vi "Actor Core.vi"(8 "error in":errorcluster, 11 "Master Controller in":refnum<class "EMS User Interface.lvclass">) -> (0 "error out":errorcluster, 3 "Actor out":refnum<class "Actor.lvclass">)   [LabVIEW 2018, in "EMS User Interface Actor.lvlib" / "EMS User Interface.lvclass"]
doc: "(<B>Filename</B>: Actor Framework.lvlib:Actor.lvclass:Actor Core.vi)\n\nReceives messages to the actor, reacts to them, and initiates any error handling that may shut the actor down.\n\nDescendant classes may override this VI to append parallel tasks for the actor to complete while it handles messages. Overrides use the Call Parent Method node."
uses:
  EMS User Interface.lvclass
  C:/Users/Administrator/Desktop/FOR GITHUB UPLOAD/LabVIEW EMS/EMS Generic Actor/EMS Generic/EMS Generic.lvclass
  C:/Program Files (x86)/National Instruments/LabVIEW 2018/vi.lib/ActorFramework/Actor/Actor.lvclass
  <vilib>/ActorFramework/Actor/Actor.lvclass
  Controls/Control Mode Tab Control.ctl
  Controls/Manual Control Tab Control.ctl
  <vilib>/ORNL/CSEISMIC DDS/CSEISMIC DDS Base/Data Types/Controls/Generation Mode.ctl
  <vilib>/ORNL/CSEISMIC DDS/CSEISMIC DDS Base/Data Types/Controls/DeviceID.ctl
  EMS Core/EMS/Controls/Microgrid State.ctl
  Utilities/Status Messaging.llb/Status Message Command.ctl
  EMS Generic Actor/EMS Generic/Controls/Device Information Cluster.ctl
  EMS Generic Actor/EMS Generic/Controls/Device State.ctl
  Controls/Listbox Columns.ctl
  EMS User Interface.lvclass/EMS User Interface.ctl
  <vilib>/ActorFramework/Actor/Actor.lvclass/Actor.ctl
  <vilib>/ActorFramework/Message Enqueuer/Message Enqueuer.lvclass/Message Enqueuer.ctl
  EMS User Interface Messages/Launch Save Status Msg/Launch Save Status Msg.lvclass/Launch Save Status Msg.ctl
  Controls/Dialog Message Selector.ctl
  EMS User Interface Messages/Call Dialog Msg/Call Dialog Msg.lvclass/Call Dialog Msg.ctl
  EMS User Interface Messages/Connect to Device Msg/Connect to Device Msg.lvclass/Connect to Device Msg.ctl
  <vilib>/ORNL/CSEISMIC DDS/CSEISMIC DDS Base/Data Types/DER_Control.ctl
  EMS Core/EMS Messages/Manual Activate Msg/Manual Activate Msg.lvclass/Manual Activate Msg.ctl
  <vilib>/ORNL/CSEISMIC DDS/CSEISMIC DDS Base/Data Types/DER_SetPointP.ctl
  EMS Core/EMS Messages/Manual Real Power Setpoint Msg/Manual Real Power Setpoint Msg.lvclass/Manual Real Power Setpoint Msg.ctl
  <vilib>/ORNL/CSEISMIC DDS/CSEISMIC DDS Base/Data Types/DER_setGenerationMode.ctl
  EMS Core/EMS Messages/Manual Generation Mode Set Msg/Manual Generation Mode Set Msg.lvclass/Manual Generation Mode Set Msg.ctl
  <vilib>/ORNL/CSEISMIC DDS/CSEISMIC DDS Base/Data Types/DER_SetPointQ.ctl
  EMS Core/EMS Messages/Manual Reactive Power Setpoint Msg/Manual Reactive Power Setpoint Msg.lvclass/Manual Reactive Power Setpoint Msg.ctl
  <vilib>/Utility/miscctls.llb/LVRowAndColumnTypeDef.ctl
  <vilib>/ORNL/CSEISMIC DDS/CSEISMIC DDS Base/Data Types/IED_Status.ctl
  <vilib>/ORNL/CSEISMIC DDS/CSEISMIC DDS Base/Data Types/Controls/Timestamp.ctl
  <vilib>/ORNL/CSEISMIC DDS/CSEISMIC DDS Base/Data Types/DER_Measurement.ctl
  <vilib>/ORNL/CSEISMIC DDS/CSEISMIC DDS Base/Data Types/SmartRelay_Measurement.ctl
  <vilib>/ORNL/CSEISMIC DDS/CSEISMIC DDS Base/Data Types/DER_Status.ctl
  <vilib>/ORNL/CSEISMIC DDS/CSEISMIC DDS Base/Data Types/Controls/DroopCurve.ctl
  <vilib>/Analysis/1siggen.llb/Ramp Pattern by Samples.vi
  <vilib>/ActorFramework/Message Enqueuer/Init from Existing Queue.vi
  <vilib>/ActorFramework/Message Enqueuer/Enqueue.vi
  EMS User Interface Messages/Reset Configuration Msg/Reset Configuration Msg.lvclass
  C:/Program Files (x86)/National Instruments/LabVIEW 2018/vi.lib/ActorFramework/Message/Message.lvclass
  EMS User Interface Messages/Launch Save Configuration Msg/Launch Save Configuration Msg.lvclass
  EMS User Interface Messages/Launch Load Configuration Msg/Launch Load Configuration Msg.lvclass
  <vilib>/ActorFramework/Stop Msg/Stop Msg.lvclass
  EMS User Interface Messages/Launch Save Status Msg/Launch Save Status Msg.lvclass
  EMS User Interface Messages/Set Default Configuration Msg/Set Default Configuration Msg.lvclass
  EMS User Interface Messages/Launch Devices to Load Dialog Msg/Launch Devices to Load Dialog Msg.lvclass
  EMS User Interface Messages/Launch VF Device Selection Dialog Msg/Launch VF Device Selection Dialog Msg.lvclass
  EMS User Interface Messages/Call Dialog Msg/Call Dialog Msg.lvclass
  EMS User Interface Messages/Automatic EMS Msg/Automatic EMS Msg.lvclass
  EMS User Interface Messages/Manual EMS Msg/Manual EMS Msg.lvclass
  EMS User Interface Messages/Start EMS Msg/Start EMS Msg.lvclass
  EMS User Interface Messages/Execute EMS Msg/Execute EMS Msg.lvclass
  EMS User Interface Messages/Transition EMS Msg/Transition EMS Msg.lvclass
  EMS User Interface Messages/Connect to Device Msg/Connect to Device Msg.lvclass
  EMS Core/EMS Messages/Manual Activate Msg/Manual Activate Msg.lvclass
  EMS Core/EMS Messages/Manual Real Power Setpoint Msg/Manual Real Power Setpoint Msg.lvclass
  EMS Core/EMS Messages/Manual Generation Mode Set Msg/Manual Generation Mode Set Msg.lvclass
  EMS Core/EMS Messages/Manual Reactive Power Setpoint Msg/Manual Reactive Power Setpoint Msg.lvclass
  Global Variables/Global Variables.vi
  <vilib>/ActorFramework/Message Priority Queue/Priority Enqueue.vi
  <vilib>/ActorFramework/Message Enqueuer/Message Enqueuer.lvclass
  EMS Generic Actor/EMS Generic/EMS Generic.lvclass
  EMS Core/EMS/EMS.lvclass
  Utilities/Status Messaging.llb/Status Messaging.lvlib
  <vilib>/ORNL/CSEISMIC DDS/CSEISMIC DDS Base/CSEISMIC DDS.lvclass
  Utilities/Password Protection/Password Protection.lvlib
  <vilib>/Analysis/NI_AALBase.lvlib
panel:
  out "DevIDs in Config":T1[](array[typedef])
  in  "Control Mode":T2
  out "Current Status Bool":bool
  out "Current State":string
  out "Current Status":string
  in  "Transition":bool
  in  "Execution":bool
  in  "Start":bool
  out "Status":string
  out "Devices":i32(listbox)
  in  "Connect":bool
  out "Manual Status":string
  in  "Device Connect":T3
  in  "Activate Device?":bool caption="Activate\nDevice?"
  in  "Write Mode":bool caption="Write\nMode"
  in  "Write Q":bool
  in  "Write P":bool
  in  "Q Setpoint (kVAR)":dbl(slide) scale=0.0..330.0
  in  "P Setpoint (kW)":dbl(slide) scale=0.0..330.0 scale format="%#.6g"
  in  "Write Activation":bool caption="Write\nActivation"
  out "P Meas":dbl[](array[numeric])
  out "Q Meas":dbl[](array[numeric])
  in  "Gen Mode":T4=enum."PQ"
  out "Active":bool
  out "Inactive":bool
  in  "Channels":i32[](listbox)
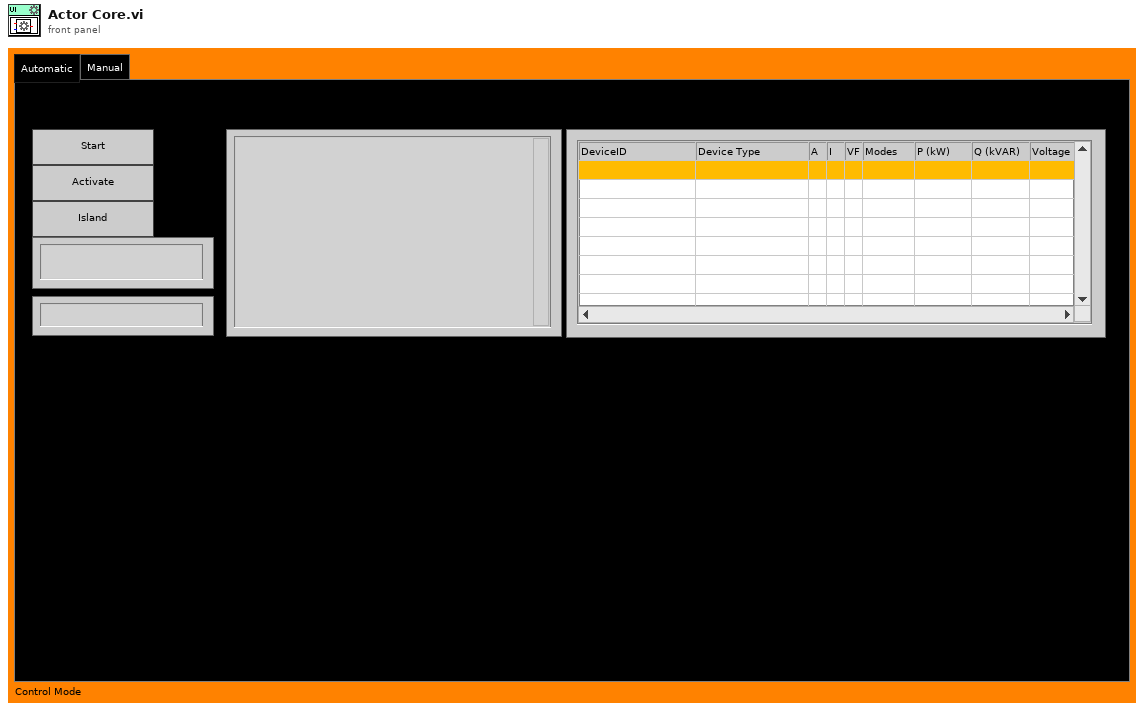
[diagram p1: front panel]
types:
  T1 = typedef "CSEISMIC DDS.lvlib/CSEISMIC DDS.lvclass/DeviceID.ctl" = string
  T2 = typedef "EMS User Interface Actor.lvlib/EMS User Interface.lvclass/Control Mode Tab Control.ctl" = enum32{"Automatic", "Manual"}
  T3 = typedef "EMS User Interface Actor.lvlib/EMS User Interface.lvclass/Manual Control Tab Control.ctl" = enum32{"Off", "Standard"}
  T4 = typedef "CSEISMIC DDS.lvlib/CSEISMIC DDS.lvclass/Generation Mode.ctl" = enum32{"Invalid", "PQ", "Droop", "PV", "PF", "VF"}
  T5 = typedef "EMS User Interface Actor.lvlib/EMS User Interface.lvclass/Listbox Columns.ctl" = cluster{"DeviceID Column":i32, "Device Type Column":i32, "Active Column":i32, "Inactive Column":i32, "VF Column":i32, "Modes Column":i32, "P_Total Column":i32, "Q_Total Column":i32, "V_Avg Column":i32, "I_Total Column":i32, "Frequency Column":i32, "P_A Column":i32, "P_B Column":i32, "P_C Column":i32, "Q_A Column":i32, "Q_B Column":i32, "Q_C Column":i32, "V_A Column":i32, "V_B Column":i32, "V_C Column":i32, "I_A Column":i32, "I_B Column":i32, "I_C Column":i32}
  T6 = typedef "EMS Generic Actor.lvlib/EMS Generic.lvclass/Device Information Cluster.ctl" = cluster{"Device State":T7, "data":variant}
  T7 = typedef "EMS Generic Actor.lvlib/EMS Generic.lvclass/Device State.ctl" = enum16{"Invalid", "Clear", "DevIDs in Config", "DevIDs on uGrid", "DevIDs not on uGrid", "Update IED_Status", "Update DER_Status", "Update DER_Measurement", "Update SmartRelay_Measurement"}
  T8 = enum32{"Invalid", "Standard", "Closed", "Hidden", "Minimized", "Maximized"}
  T9 = typedef "Status Messaging.lvlib/Status Message Command.ctl" = enum16{"Write", "Obtain", "Kill"}
  T10 = typedef "EMS Core.lvlib/EMS.lvclass/Microgrid State.ctl" = enum16{"Discovery", "Commissioning", "Activation", "Blackstart", "OnGrid", "OffGrid", "Island", "Resynchronization", "Manual", "Shutdown", "Stop"}
  T11 = typedef "EMS User Interface Actor.lvlib/EMS User Interface.lvclass/Master Controller User Events.ctl" = cluster{"Current State":refnum<user-event>, "Current Status":refnum<user-event>, "Device List":refnum<user-event>, "P Meas":refnum<user-event>, "Q Meas":refnum<user-event>, "P Set Max":refnum<user-event>, "Q Set Max":refnum<user-event>, "IED_Status":refnum<user-event>, "Device State Information":refnum<user-event>}
  T12 = typedef "EMS User Interface Actor.lvlib/EMS User Interface.lvclass/Dialog Message Selector.ctl" = enum16{"Nominal Voltage", "Nominal Frequency", "Optimization Parameters"}
  T13 = typedef "CSEISMIC DDS.lvlib/CSEISMIC DDS.lvclass/DER_Control.ctl" = cluster{"DeviceID":T1, "Activate":bool, "Deactivate":bool}
  T14 = typedef "CSEISMIC DDS.lvlib/CSEISMIC DDS.lvclass/DER_SetPointP.ctl" = cluster{"DeviceID":T1, "RealPower (kW)":dbl[]}
  T15 = typedef "CSEISMIC DDS.lvlib/CSEISMIC DDS.lvclass/DER_setGenerationMode.ctl" = cluster{"DeviceID":T1, "Mode":T4}
  T16 = typedef "CSEISMIC DDS.lvlib/CSEISMIC DDS.lvclass/DER_SetPointQ.ctl" = cluster{"DeviceID":T1, "ReactivePower (kVAR)":dbl[]}
  T17 = enum8{"Enabled", "Disabled", "Disabled and Grayed Out"}
  T18 = typedef "LVRectTypeDef.ctl" = cluster{"Left":i16, "Top":i16, "Right":i16, "Bottom":i16}
  T19 = typedef "LVRowAndColumnTypeDef.ctl" = cluster{"Row":i32, "Column":i32}
  T20 = typedef "CSEISMIC DDS.lvlib/CSEISMIC DDS.lvclass/IED_Status.ctl" = cluster{"DeviceID":T1, "Timestamp":T21, "MicrogridID":u8, "Active":bool, "Inactive":bool, "Error":i32, "Fault":bool, "ErrorString":string}
  T21 = typedef "CSEISMIC DDS.lvlib/CSEISMIC DDS.lvclass/Timestamp.ctl" = cluster{"Seconds":u64, "Remainder":u64}
  T22 = typedef "CSEISMIC DDS.lvlib/CSEISMIC DDS.lvclass/DER_Measurement.ctl" = cluster{"DeviceID":T1, "Voltage":dbl[], "Current":dbl[], "RealPower":dbl[], "ReactivePower":dbl[], "LineConfig":u8[], "Frequency":dbl}
  T23 = typedef "CSEISMIC DDS.lvlib/CSEISMIC DDS.lvclass/SmartRelay_Measurement.ctl" = cluster{"DeviceID":T1, "PrimaryVoltage":dbl[], "SecondaryVoltage":dbl[], "Current":dbl[], "RealPower":dbl[], "ReactivePower":dbl[], "LineConfig":u8[], "Frequency":dbl}
  T24 = typedef "CSEISMIC DDS.lvlib/CSEISMIC DDS.lvclass/DER_Status.ctl" = cluster{"DeviceID":T1, "VFControl":bool, "PControl":bool, "QControl":bool, "PFControl":bool, "PVControl":bool, "Droop":bool, "Unbalanced":bool, "MicrogridVF":bool, "RealDroop(kW)":T25, "ReactiveDroop(kVar)":T25}
  T25 = typedef "CSEISMIC DDS.lvlib/CSEISMIC DDS.lvclass/DroopCurve.ctl" = cluster{"XMin":dbl, "XMax":dbl, "YMin":dbl, "YMax":dbl}
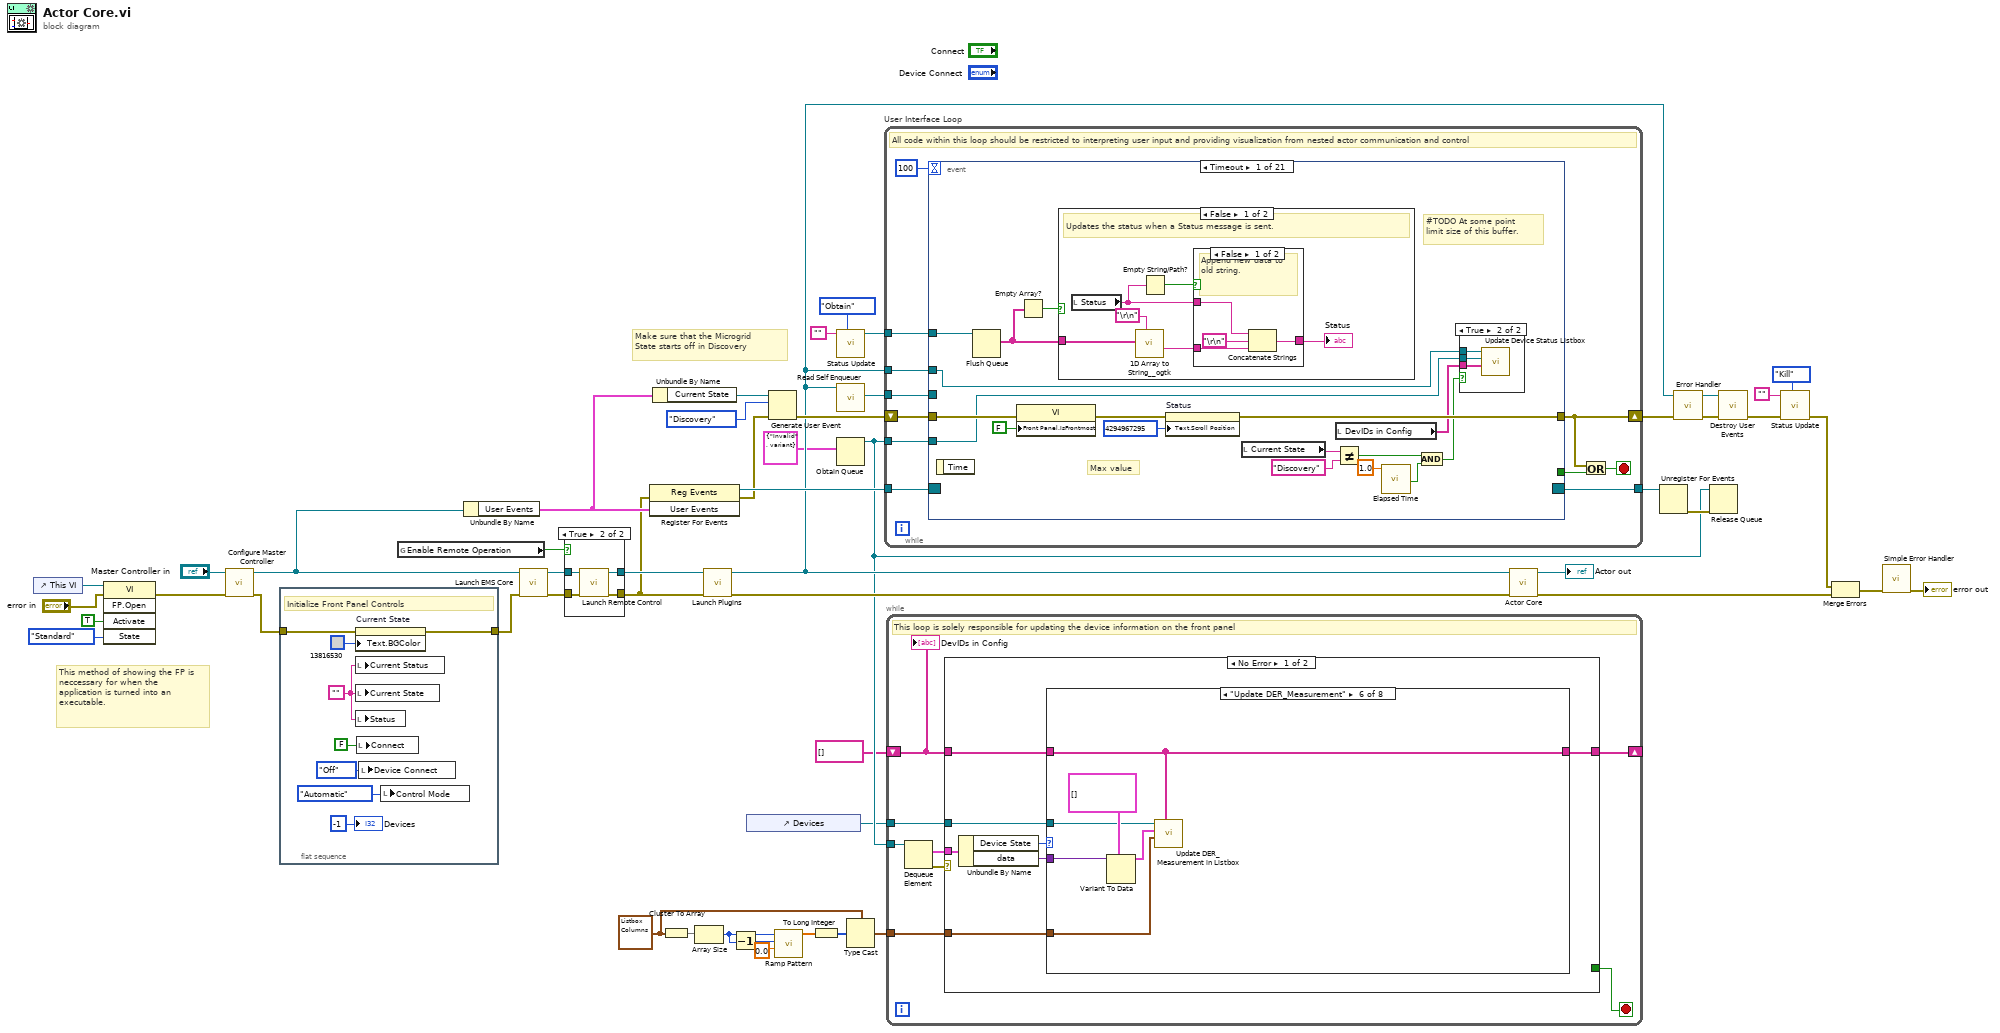
[diagram p0: block diagram]
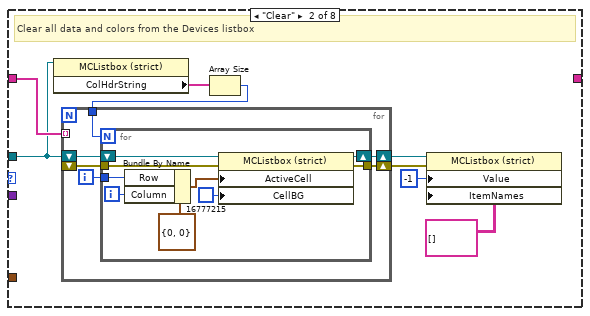
[diagram p3: hidden frame]
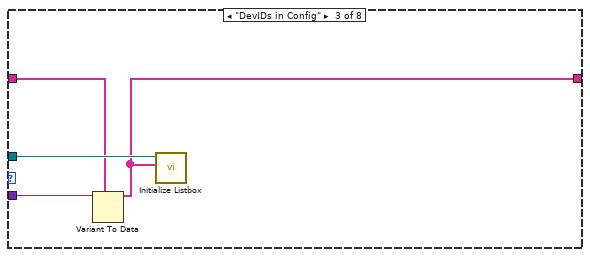
[diagram p4: hidden frame]
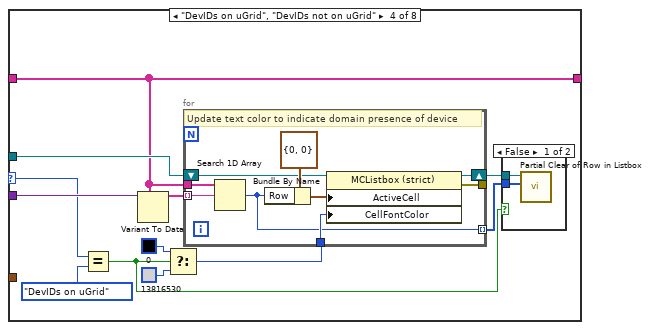
[diagram p5: hidden frame]
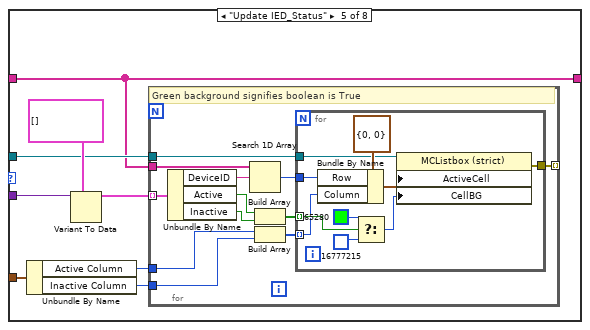
[diagram p7: hidden frame]
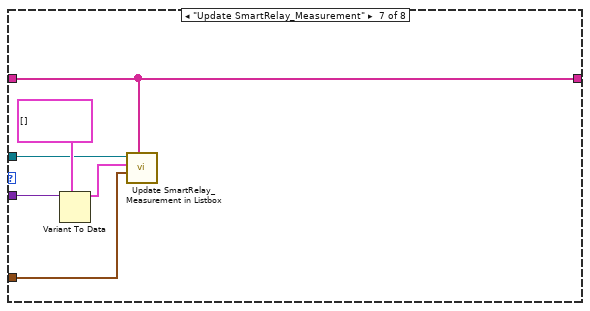
[diagram p8: hidden frame]
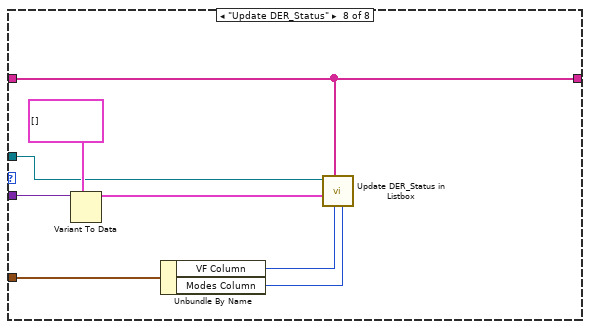
[diagram p9: hidden frame]
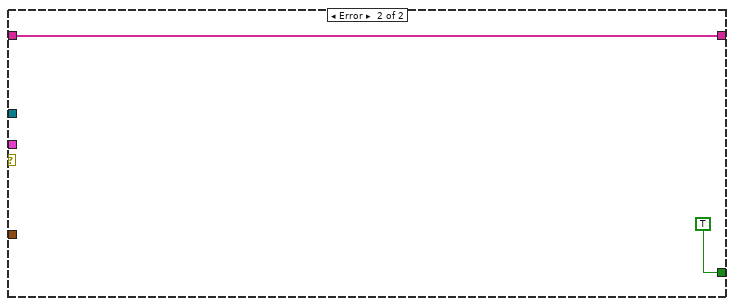
[diagram p10: hidden frame]
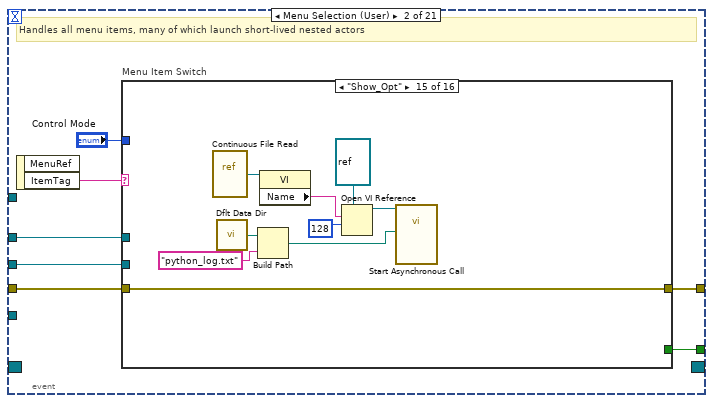
[diagram p15: hidden frame]
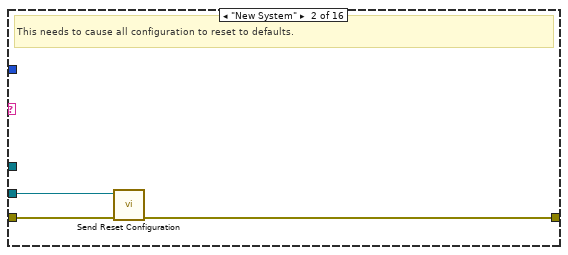
[diagram p17: hidden frame]
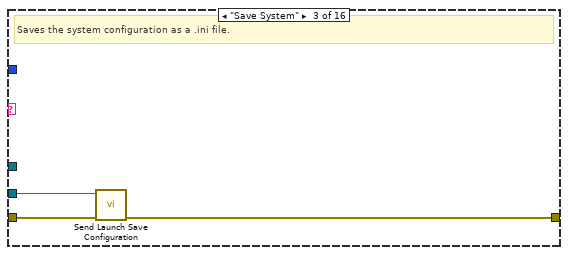
[diagram p18: hidden frame]
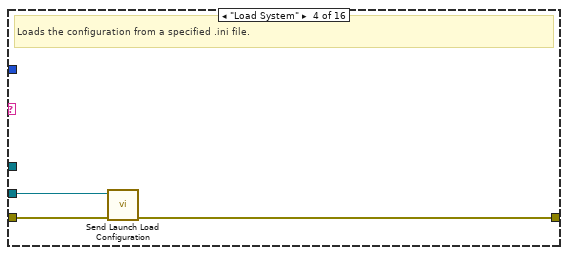
[diagram p19: hidden frame]
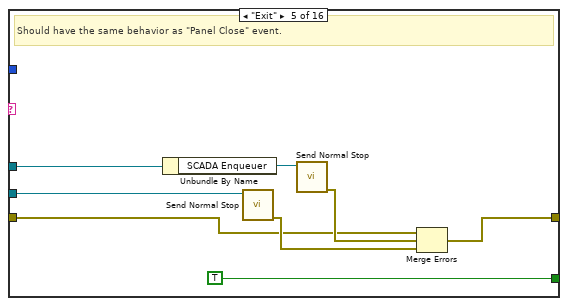
[diagram p20: hidden frame]
diagram:
  w1 = T5 {"DeviceID Column"=0, "Device Type Column"=0, "Active Column"=0, "Inactive Column"=0, "VF Column"=0, "Modes Column"=0, "P_Total Column"=0, "Q_Total Column"=0, "V_Avg Column"=0, "I_Total Column"=0, "Frequency Column"=0, "P_A Column"=0, "P_B Column"=0, "P_C Column"=0, "Q_A Column"=0, "Q_B Column"=0, "Q_C Column"=0, "V_A Column"=0, "V_B Column"=0, "V_C Column"=0, "I_A Column"=0, "I_B Column"=0, "I_C Column"=0} ("DER_Meas Listbox Columns")
  # "Make sure that the Microgrid State starts off in Discovery"
  # "This method of showing the FP is neccessary for when the application is turned into an executable."
  n1 = control-ref of="This VI"() -> (w34:refnum<vi>)
  n2 = invoke class="VI" method="FP.Open"(reference=w34, error in="error in", "Activate"=TRUE ("Activate?"), "State"=T8."Standard") -> (error out=w30:errorcluster)  [unwired: 1 in, 4 out]
  n3 = call "Configure Master Controller.vi"("error in"=w30, "EMS Generic in"="Master Controller in") -> ("error out"=w41:errorcluster, "EMS Generic out"=w42:refnum<class "EMS User Interface.lvclass">)  [unwired: 8 in]
  n4 = flat-sequence {
    tunnel: w41 -> [w57]
    tunnel: [w56] -> w47
    frame #0 {
      w59 = ""
      # "Initialize Front Panel Controls"
      n5 = property on="Current State" class="Str"(error in=w57, "Text.BGColor"=u32 13816530) -> (error out=w56:errorcluster)  [unwired: 1 in, 1 out]
      n6 = local write "Current Status"(w59) -> ()
      n7 = local write "Current State"(w59) -> ()
      n8 = local write "Status"(w59) -> ()
      n9 = local write "Connect"(FALSE ("Connect")) -> ()
      n10 = local write "Device Connect"(Manual_Control_Tab_Control."Off" ("Device Connect")) -> ()
      n11 = local write "Control Mode"(Control_Mode_Tab_Control."Automatic" ("Control Mode")) -> ()
      "Devices" <- -1 ("Devices")
    }
  }
  n12 = global read "Global Variables.vi" "Enable Remote Operation"() -> (w18:bool)
  n13 = Unbundle By Name(w42) -> ("User Events"=w45:T11)
  n14 = call "Launch EMS Core.vi"("error in"=w47, "Master Controller in"=w42) -> ("error out"=w19:errorcluster, "Master Controller out"=w20:refnum<class "EMS User Interface.lvclass">)  [unwired: 8 in]
  n15 = case shown="True" w18 {
    tunnel: w20 -> [w61 w65]
    tunnel: [w61 w64] -> w17
    tunnel: w19 -> [w60 w63]
    tunnel: [w60 w62] -> w16
    frame False {
    }
    frame True {
      n16 = call "Launch Remote Control.vi"("error in"=w63, "Master Controller in"=w65) -> ("error out"=w62:errorcluster, "Master Controller out"=w64:refnum<class "EMS User Interface.lvclass">)  [unwired: 8 in]
    }
  }
  n17 = register-events(error in=w16, w45) -> (reference out=w50:refnum<event-registration>, error out=w46:errorcluster)  [unwired: 1 in]
  n18 = Unbundle By Name(w45) -> ("Current State"=w44:refnum<user-event>)
  n19 = Cluster To Array(cluster=w1) -> (array=w5:i32[])
  n20 = Array Size(array=w5) -> (size(s)=w6:i32)
  n21 = call "Launch Plugins.vi"("error in"=w16, "Master Controller in"=w17) -> ("error out"=w14:errorcluster, "Master Controller out"=w15:refnum<class "EMS User Interface.lvclass">)  [unwired: 8 in]
  n22 = Decrement(x=w6) -> (x-1=w8:i32)
  n23 = control-ref of="Devices"() -> (w10:refnum<vi>)
  n24 = Generate User Event(user event=w44, event data cluster=Microgrid_State."Discovery" ("event data"), error in=w46) -> (error out=w27:errorcluster)  [unwired: 1 in, 1 out]
  n25 = call-poly <vilib>:"Ramp Pattern.vi"("start"=0.0, "end"=w8, "samples"=w6) -> ("Ramp Pattern"=w4:dbl[])  [unwired: 7 in, 1 out]
  n26 = To Long Integer(number=w4) -> (32bit integer=w3:i32[])
  n27 = call "Status Update.vi"("Command (Write)"=Status_Message_Command."Obtain", "Status Update"="") -> ("queue out"=w38:refnum<queue>)  [unwired: 8 in, 1 out]
  n28 = call <vilib>:"Read Self Enqueuer.vi"("Actor"=w15) -> ("Self Enqueuer"=w48:refnum<class "Message Enqueuer.lvclass">)  [unwired: 10 in]
  n29 = Obtain Queue(element data type=T6 {"Device State"=enum."Invalid", "data"=variant} ("Device State Information")) -> (queue out=w11:refnum<queue>)  [unwired: 4 in, 2 out]
  n30 = Type Cast(type=w1, x=w3) -> (*(type *) &x=w2:T5)
  n31 = while "User Interface Loop" {
    shift-right: [w69] -> w23
    shift-left: w27 -> [w76]
    tunnel: w50 -> [w75]
    tunnel: [w74] -> w49
    tunnel: w48 -> [w73]
    tunnel: w38 -> [w72]
    tunnel: w15 -> [w70]
    tunnel: w11 -> [w66]
    stop <- w67 stop-if-true
    # "All code within this loop should be restricted to interpreting user input and providing visualization from nested actor communication and control"
    n32 = event shown="[0] Timeout" {
      selector: w75 -> [_ _ _ _ _ _ _ _ _ _ _ _ _ _ _ _ _ _ _ _ _]
      dyn-events: [_ _ _ _ _ _ _ _ _ _ _ _ _ _ _ _ _ _ _ _ _] -> w74
      timeout: 100 -> [_ _ _ _ _ _ _ _ _ _ _ _ _ _ _ _ _ _ _ _ _]
      tunnel: w76 -> [w92 w112 w210 w213 w222 w230 w238 w274 w292 w313 w330 _ w360 _ w491 _ _ w506 w510 _ w516]
      tunnel: [w93 w111 w209 w212 w223 w229 w237 w273 w291 w312 w329 _ w362 _ w478 _ _ w505 w508 _ w513] -> w69
      tunnel: [_ w110 _ _ _ _ _ _ _ _ _ _ _ _ _ _ _ _ _ _ TRUE ("Discard?")] -> w68
      tunnel: w73 -> [_ w113 w211 w214 w224 w231 w239 _ _ _ _ _ _ _ _ _ _ _ _ _ w517]
      tunnel: w72 -> [w91 _ _ _ _ _ _ _ _ _ _ _ _ _ _ _ _ _ _ _ _]
      tunnel: w70 -> [w83 w108 _ _ _ _ _ w272 w293 w314 w328 _ w357 _ _ _ _ _ _ _ w519]
      tunnel: w66 -> [w84 _ _ _ _ _ _ _ _ _ _ w350 w356 _ _ _ _ _ _ _ _]
      event Timeout {
        # "Max value"
        # "#TODO At some point limit size of this buffer."
        n33 = event-data() -> ()  [unwired: 1 in, 1 out]
        n34 = Flush Queue(queue=w91) -> (remaining elements=w87:string[])  [unwired: 1 in, 2 out]
        n35 = property class="VI"(error in=w92, "Front Panel.IsFrontmost"=FALSE ("Front Panel Window:Is Frontmost")) -> (error out=w89:errorcluster)  [unwired: 1 in, 1 out]
        n36 = Empty Array?(array=w87) -> (empty?=w86:bool)
        n37 = case shown="False" w86 {
          tunnel: w87 -> [w99 _]
          frame False {
            # "Updates the status when a Status message is sent."
            n38 = local read "Status"() -> (w100:string)
            n39 = call <userlib>:"1D Array to String__ogtk.vi"("delimiter (Tab)"="\r\n", "Array of Strings"=w99) -> ("delimited string"=w97:string)  [unwired: 9 in]
            n40 = Empty String/Path?(string/path=w100) -> (empty?=w101:bool)
            n41 = case shown="False" w101 {
              tunnel: [w106 w107] -> w102
              tunnel: w97 -> [w105 w107]
              tunnel: w100 -> [w103 _]
              frame False {
                # "Append new data to old string."
                n42 = Concatenate Strings(w103, "\r\n", w105) -> (w106:string)
              }
              frame True {
                # "Set new data as string."
              }
            }
            "Status" <- w102
          }
          frame True {
          }
        }
        n43 = property on="Status" class="Str"(error in=w89, "Text.Scroll Position"=u32 4294967295) -> (error out=w93:errorcluster)  [unwired: 1 in, 1 out]
        n44 = local read "Current State"() -> (w81:string)
        n45 = local read "DevIDs in Config"() -> (w82:T1[])
        n46 = Not Equal?(x=w81, y="Discovery") -> (x != y?=w79:bool)
        n47 = call "Elapsed Time"("Time Target (s)"=1.0) -> ("Time has Elapsed"=w78:bool)  [unwired: 11 in, 7 out]
        n48 = And(x=w79, y=w78) -> (x .and. y?=w77:bool)
        n49 = case shown="True" w77 {
          tunnel: w84 -> [_ w96]
          tunnel: w83 -> [_ w95]
          tunnel: w82 -> [_ w94]
          frame False {
          }
          frame True {
            n50 = call "Update Device Status Listbox.vi"("DeviceIDs"=w94, "queue in"=w96, "EMS User Interface in"=w95) -> ()  [unwired: 9 in]
          }
        }
      }
      event Menu Selection (User) {
        # "Handles all menu items, many of which launch short-lived nested actors"
        n51 = event-data() -> ("ItemTag"=w114:string)  [unwired: 1 in, 1 out]
        n52 = case "Menu Item Switch" shown="\"Show_Opt\"" w114 {
          tunnel: w113 -> [_ w118 w119 w123 w126 w134 _ w141 w144 w147 w149 w153 w156 w176 _ w205]
          tunnel: w112 -> [w115 w117 w121 w124 w128 w136 w138 w140 w143 w146 w151 w155 w160 w180 w204 w207]
          tunnel: [w115 w116 w120 w122 w127 w135 w138 w139 w142 w145 w150 w154 w159 w179 w204 w206] -> w111
          tunnel: [_ _ _ _ TRUE ("Discard?") _ _ _ _ _ _ _ _ _ _ _] -> w110
          tunnel: "Control Mode" -> [_ _ _ _ _ _ _ _ _ _ _ _ w158 w178 _ _]
          tunnel: w108 -> [_ _ _ _ w125 _ _ _ _ _ _ _ _ _ _ _]
          frame "False", Default {
            # "Do nothing for unconfigured menu items"
          }
          frame "New System" {
            # "This needs to cause all configuration to reset to defaults."
            n53 = call "Send Reset Configuration.vi"("error in (no error)"=w117, "Message Enqueuer"=w118) -> ("error out"=w116:errorcluster)  [unwired: 8 in, 1 out]
          }
          frame "Save System" {
            # "Saves the system configuration as a .ini file."
            n54 = call "Send Launch Save Configuration.vi"("error in (no error)"=w121, "Message Enqueuer"=w119) -> ("error out"=w120:errorcluster)  [unwired: 8 in, 1 out]
          }
          frame "Load System" {
            # "Loads the configuration from a specified .ini file."
            n55 = call "Send Launch Load Configuration.vi"("error in (no error)"=w124, "Message Enqueuer"=w123) -> ("error out"=w122:errorcluster)  [unwired: 8 in, 1 out]
          }
          frame "Exit" {
            # "Should have the same behavior as \"Panel Close\" event."
            n56 = Unbundle By Name(w125) -> ("SCADA Enqueuer"=w129:refnum<class "Message Enqueuer.lvclass">)
            n57 = call <vilib>:"Send Normal Stop.vi"("Message Enqueuer"=w126) -> ("error out"=w131:errorcluster)  [unwired: 10 in]
            n58 = call <vilib>:"Send Normal Stop.vi"("Message Enqueuer"=w129) -> ("error out"=w130:errorcluster)  [unwired: 10 in]
            n59 = Merge Errors(w128, w130, w131) -> (w127:errorcluster)
          }
          frame "Save Status History" {
            # "Saves the Status text box to a text file."
            n60 = local read "Status"() -> (w133:string)
            n61 = call "Send Launch Save Status.vi"("error in (no error)"=w136, "Status"=w133, "Message Enqueuer"=w134) -> ("error out"=w135:errorcluster)  [unwired: 7 in, 1 out]
          }
          frame "Clear Status History" {
            # "Clears the Status text box."
            n62 = local write "Status"("") -> ()
          }
          frame "DEFAULT" {
            # "Set the current configuration file as the default configuration file."
            n63 = call "Send Set Default Configuration.vi"("error in (no error)"=w140, "Message Enqueuer"=w141) -> ("error out"=w139:errorcluster)  [unwired: 8 in, 1 out]
          }
          frame "Devices to Load" {
            # "Launches a dialog box that allows the user to choose which available device to use in the system."
            n64 = call "Send Launch Devices to Load Dialog.vi"("error in (no error)"=w143, "Message Enqueuer"=w144) -> ("error out"=w142:errorcluster)  [unwired: 8 in, 1 out]
          }
          frame "V/F Device" {
            # "Launches a dialog box that allows the user to choose which available device to use in the system."
            n65 = call "Send Launch VF Device Selection Dialog.vi"("error in (no error)"=w146, "Message Enqueuer"=w147) -> ("error out"=w145:errorcluster)  [unwired: 8 in, 1 out]
          }
          frame "Nominal Frequency" {
            # "Launch a subactor to set the nominal frequency"
            n66 = call "Send Call Dialog.vi"("error in (no error)"=w151, "Dialog"=Dialog_Message_Selector."Nominal Frequency", "Message Enqueuer"=w149) -> ("error out"=w150:errorcluster)  [unwired: 7 in, 1 out]
          }
          frame "Nominal Voltage" {
            # "Launches a subactor to set Nominal Voltage"
            n67 = call "Send Call Dialog.vi"("error in (no error)"=w155, "Dialog"=Dialog_Message_Selector."Nominal Voltage", "Message Enqueuer"=w153) -> ("error out"=w154:errorcluster)  [unwired: 7 in, 1 out]
          }
          frame "Automatic" {
            # "Change the visible area and window position for Automatic Control Mode"
            n68 = case shown="\"Manual\"" w158 {
              tunnel: w160 -> [w161 w164]
              tunnel: [w161 w170] -> w159
              tunnel: w156 -> [_ w165]
              frame "Automatic", Default {
                # "If it's already Automatic/Normal, do nothing"
              }
              frame "Manual" {
                # "Make sure that the current control mode is Manual"
                n69 = control-ref of="This VI"() -> (w166:refnum<vi>)
                n70 = call "Send Automatic EMS.vi"("error in (no error)"=w164, "Message Enqueuer"=w165) -> ("error out"=w163:errorcluster)  [unwired: 8 in, 1 out]
                n71 = property class="VI"(reference=w166, error in=w163) -> (reference out=w169:refnum<vi>, error out=w171:errorcluster, "Front Panel.PanelBounds"=w168:T18)
                n72 = in-place {
                  n73 = in-place-cluster #1(w168) -> ("Right"=w175:i16)
                  n74 = Add(x=w175, y=i16 -25) -> (x+y=w173:i16)
                  n75 = in-place-cluster #1("Right"=w173) -> (w167:T18)
                }
                n76 = local read "Connect"() -> (w162:bool)
                n77 = case shown="True" w162 {
                  frame False {
                  }
                  frame True {
                    n78 = property on="Connect" class="Bool (strict)"("Val(Sgnl)"=FALSE ("Connect")) -> ()  [unwired: 2 in, 2 out]
                  }
                }
                n79 = property class="VI"(reference=w169, error in=w171, "Front Panel.PanelBounds"=w167) -> (error out=w170:errorcluster)  [unwired: 1 out]
              }
            }
            n80 = local write "Control Mode"(Control_Mode_Tab_Control."Automatic" ("Control Mode")) -> ()
          }
          frame "Manual" {
            # "Change the visible area and window position for Manual Control Mode"
            n81 = case shown="\"Automatic\"" w178 {
              tunnel: w180 -> [w185 w195]
              tunnel: [w190 w195] -> w179
              tunnel: w176 -> [w186 _]
              frame "Automatic" {
                # "Make sure that the current control mode is Normal/Automatic. Adjust the window width bigger and send the message to put the EMS into the Stop state if neccessary."
                n82 = control-ref of="This VI"() -> (w183:refnum<vi>)
                n83 = call "Send Manual EMS.vi"("error in"=w185, "Message Enqueuer"=w186) -> ("error out"=w184:errorcluster)  [unwired: 8 in, 1 out]
                n84 = local write "Connect"(FALSE ("Connect")) -> ()
                n85 = local write "Manual Status"("") -> ()
                n86 = property class="VI"(reference=w183, error in=w184) -> (reference out=w189:refnum<vi>, error out=w191:errorcluster, "Front Panel.PanelBounds"=w188:T18)
                n87 = in-place {
                  n88 = in-place-cluster #2(w188) -> ("Right"=w194:i16)
                  n89 = Add(x=w194, y=i16 25) -> (x+y=w192:i16)
                  n90 = in-place-cluster #2("Right"=w192) -> (w187:T18)
                }
                n91 = property class="VI"(reference=w189, error in=w191, "Front Panel.PanelBounds"=w187) -> (error out=w190:errorcluster)  [unwired: 1 out]
              }
              frame "Manual", Default {
                # "If it's already Manual, do nothing"
              }
            }
            n92 = local write "Control Mode"(Control_Mode_Tab_Control."Manual" ("Control Mode")) -> ()
          }
          frame "Show_Opt" {
            n93 = vi-ref "Continuous File Read.vi"() -> (w197:refnum<vi>)
            n94 = call <vilib>:"Dflt Data Dir.vi"() -> ("App:Default Data Directory"=w203:path)
            n95 = Build Path(base path=w203, name or relative path="python_log.txt") -> (appended path=w198:path)
            n96 = property class="VI"(reference=w197) -> ("Name"=w196:string)  [unwired: 1 in, 2 out]
            n97 = Open VI Reference(type specifier VI Refnum (for type only)=refnum<vi> refnum, vi path=w196, options=128) -> (vi reference=w199:refnum<vi>)  [unwired: 3 in, 1 out]
            n98 = call-by-ref "Start Asynchronous Call"(reference=w199, "file path"=w198) -> ()  [unwired: 11 in, 3 out]
          }
          frame "Opt_Params" {
            n99 = call "Send Call Dialog.vi"("error in (no error)"=w207, "Dialog"=Dialog_Message_Selector."Optimization Parameters", "Message Enqueuer"=w205) -> ("error out"=w206:errorcluster)  [unwired: 7 in, 1 out]
          }
        }
      }
      event "Start": Value Change {
        # "React to a vlaue change in the START button. This is context-specific and reacts differently based on the Microgrid state"
        n100 = event-data() -> ()  [unwired: 1 in, 1 out]
        n101 = call "Send Start EMS.vi"("error in (no error)"=w210, "Message Enqueuer"=w211) -> ("error out"=w209:errorcluster)  [unwired: 8 in, 1 out]
      }
      event "Execution": Value Change {
        # "React to a vlaue change in the EXECUTION button. This is context-specific and reacts differently based on the Microgrid state"
        n102 = event-data() -> ()  [unwired: 1 in, 1 out]
        n103 = call "Send Execute EMS.vi"("error in (no error)"=w213, "Message Enqueuer"=w214) -> ("error out"=w212:errorcluster)  [unwired: 8 in, 1 out]
      }
      event "Transition": Value Change {
        # "React to a vlaue change in the TRANSITION button. This is context-specific and reacts differently based on the Microgrid state"
        n104 = event-data() -> ()  [unwired: 1 in, 1 out]
        n105 = call <vilib>:"Application Directory.vi"() -> ("Application Directory"=w218:path)
        n106 = Build Path(base path=w218, name or relative path="Configuration") -> (appended path=w217:path)
        n107 = Build Path(base path=w217, name or relative path="EMS-config.ini") -> (appended path=w215:path)
        n108 = call "Password Protection.vi"("error in"=w222, "configuration file path"=w215) -> ("error out"=w221:errorcluster, "Validated?"=w220:bool)  [unwired: 8 in]
        n109 = case shown="True" w220 {
          tunnel: w224 -> [_ w228]
          tunnel: [w225 w227] -> w223
          tunnel: w221 -> [w225 w226]
          frame False {
          }
          frame True {
            n110 = call "Send Transition EMS.vi"("error in (no error)"=w226, "Message Enqueuer"=w228) -> ("error out"=w227:errorcluster)  [unwired: 8 in, 1 out]
          }
        }
      }
      event "Channels": Value Change {
        # "Solely for disconnecting the last device when it is either deselected or another device is selected"
        n111 = event-data() -> ()  [unwired: 1 in, 1 out]
        n112 = local read "Connect"() -> (w232:bool)
        n113 = case "Device Connected?" shown="True" w232 {
          tunnel: w231 -> [_ _]
          tunnel: w230 -> [w233 w236]
          tunnel: [w233 w235] -> w229
          frame False {
            # "Not connected to anything, so do nothing."
          }
          frame True {
            # "Disconnect device, we use the value change (signaling) to execute the event case for Connect Value Change."
            n114 = property on="Connect" class="Bool (strict)"(error in=w236, "Val(Sgnl)"=FALSE ("Connect")) -> (error out=w235:errorcluster)  [unwired: 1 in, 1 out]
          }
        }
      }
      event "Connect": Value Change {
        # "Connect to selected device, making a link to bringing back measurements, status, and info and allowing setting setpoints"
        n115 = event-data() -> ("NewVal"=w241:bool)  [unwired: 1 in]
        n116 = case "Connect Device?" shown="True" w241 {
          tunnel: "Channels" -> [_ w262]
          tunnel: w239 -> [w246 w260]
          tunnel: w238 -> [w245 w261]
          tunnel: [w244 w259] -> w237
          frame False {
            # "Disconnect the device. This should put the Microgrid into the Stop state, that will move into Device Discovery."
            n117 = call "Send Start EMS.vi"("error in (no error)"=w245, "Message Enqueuer"=w246) -> ("error out"=w244:errorcluster)  [unwired: 8 in, 1 out]
            n118 = local write "Manual Status"("") -> ()
            n119 = local write "Device Connect"(Manual_Control_Tab_Control."Off" ("Device Connect Tab")) -> ()
          }
          frame True {
            # "hide certain controls when manual device is PCC"
            # "Connect to the device. This puts SCADA and the Microgird into a Manual Control State"
            n120 = for {
              tunnel: w262 -> [w265] mode=indexing
              shift-right: [w267] -> _
              shift-left: w260 -> [w269]
              shift-right: [w268] -> w259
              shift-left: w261 -> [w270]
              tunnel: [w263] -> w253 mode=indexing
              # "For now, this should only run once"
              n121 = property on="Channels" class="MCListbox (strict)"() -> ("ItemNames"=w266:string[][])  [unwired: 2 in, 2 out]
              n122 = Index Array(array=w266, index (row)=w265, index (col)=3 ("disabled index (col)")) -> (element=w263:string)
              n123 = call "Send Connect to Device.vi"("error in (no error)"=w270, "DeviceID"=w263, "Message Enqueuer"=w269) -> ("error out"=w268:errorcluster, "Message Enqueuer out"=w267:refnum<class "Message Enqueuer.lvclass">)  [unwired: 7 in]
            }
            n124 = call "Determine Device Types.vi"("DeviceIDs"=w253) -> ("Device Classes"=w252:string[])  [unwired: 9 in]
            n125 = call <userlib>:"1D Array to String__ogtk.vi"("delimiter (Tab)"=",", "Array of Strings"=w253) -> ("delimited string"=w255:string)  [unwired: 9 in]
            n126 = Format Into String(format string="Connected: %s", w255) -> (resulting string=→"Manual Status":string)  [unwired: 2 in, 1 out]
            n127 = Search 1D Array(1D array=w252, element="PCC") -> (index of element=w250:i32)  [unwired: 1 in]
            n128 = Less Than 0?(x=w250) -> (x < 0?=w248:bool)
            n129 = local write "Device Connect"(Manual_Control_Tab_Control."Standard" ("Device Connect Tab")) -> ()
            n130 = control-ref of="This VI"() -> (w249:refnum<vi>)
            n131 = call "Set Visibility of Select Manual Controls.vi"("Visible (F)"=w248, "Control Names"=string[] ["P Setpoint (kW)", "Write P", "Write Mode", "Gen Mode", "Write Q", "Q Setpoint (kVAR)"], "VI in"=w249) -> ()  [unwired: 9 in]
          }
        }
      }
      event "Write Activation": Value Change {
        # "#TODO Move some of this code into a message to make sure it only runs while the microgrid is in manual mode"
        # "This event should only execute if the Microgrid is in Manual Mode and a Device is connected"
        n132 = event-data() -> ()  [unwired: 1 in, 1 out]
        n133 = local read "Device Connect"() -> (w275:T3)
        n134 = case "Device Connection Status?" shown="\"Standard\"" w275 {
          tunnel: w274 -> [w276 w287]
          tunnel: [w276 w286] -> w273
          tunnel: w272 -> [_ w289]
          tunnel: "Activate Device?" -> [_ w277]
          frame "Off", Default {
            # "do nothing"
          }
          frame "Standard" {
            # "Only allow activation or deactivation of device while connected"
            n135 = Unbundle By Name(w289) -> ("SCADA Enqueuer"=w288:refnum<class "Message Enqueuer.lvclass">)
            n136 = property on="Channels" class="MCListbox (strict)"() -> ("ItemNames"=w283:string[][], "Value"=w284:i32[])  [unwired: 2 in, 2 out]
            n137 = Index Array(array=w284) -> (element=w285:i32)  [unwired: 1 in]
            n138 = Index Array(array=w283, index (row)=w285, index (col)=3 ("disabled index (col)")) -> (element=w280:string)
            n139 = Not(x=w277) -> (.not. x?=w278:bool)
            n140 = Bundle By Name(cluster=T13 {"DeviceID"="", "Activate"=FALSE, "Deactivate"=FALSE} ("DER_Control"), "Activate"=w277, "Deactivate"=w278, "DeviceID"=w280) -> (w279:T13)
            n141 = call "Send Manual Activate.vi"("error in (no error)"=w287, "DER_Control"=w279, "Message Enqueuer"=w288) -> ("error out"=w286:errorcluster)  [unwired: 7 in, 1 out]
          }
        }
      }
      event "Write P": Value Change {
        # "#TODO Move some of this code into a message to make sure it only runs while the microgrid is in manual mode"
        # "Manually send a Real Power setpoint to the connected device."
        n142 = event-data() -> ()  [unwired: 1 in, 1 out]
        n143 = local read "Device Connect"() -> (w290:T3)
        n144 = case "Device Connection Status" shown="\"Standard\"" w290 {
          tunnel: w293 -> [_ w299]
          tunnel: w292 -> [w294 w296]
          tunnel: [w294 w295] -> w291
          frame "Off", Default {
            # "Do nothing"
          }
          frame "Standard" {
            # "Turn the single setpoint into a 3-phase setpoint, take the active DeviceID and send the message"
            n145 = Unbundle By Name(w299) -> ("SCADA Enqueuer"=w298:refnum<class "Message Enqueuer.lvclass">)
            n146 = property on="Channels" class="MCListbox (strict)"() -> ("ItemNames"=w308:string[][], "Value"=w309:i32[])  [unwired: 2 in, 2 out]
            n147 = Index Array(array=w309) -> (element=w310:i32)  [unwired: 1 in]
            n148 = Divide(x="P Setpoint (kW)", y=3.0) -> (x/y=w303:dbl)
            n149 = Initialize Array(w303, 3 ("dimension size")) -> (w300:dbl[])
            n150 = Index Array(array=w308, index (row)=w310, index (col)=3 ("disabled index (col)")) -> (element=w301:string)
            n151 = Bundle By Name(cluster=T14 {"DeviceID"="", "RealPower (kW)"=[]} ("DER_SetPointP"), "RealPower (kW)"=w300, "DeviceID"=w301) -> (w297:T14)
            n152 = call "Send Manual Real Power Setpoint.vi"("error in (no error)"=w296, "DER_SetPointP"=w297, "Message Enqueuer"=w298) -> ("error out"=w295:errorcluster)  [unwired: 7 in, 1 out]
          }
        }
      }
      event "Write Mode": Value Change {
        # "#TODO Move some of this code into a message to make sure it only runs while the microgrid is in manual mode"
        # "Manually send a Real Power setpoint to the connected device."
        n153 = event-data() -> ()  [unwired: 1 in, 1 out]
        n154 = local read "Device Connect"() -> (w311:T3)
        n155 = case "Device Connection Status" shown="\"Standard\"" w311 {
          tunnel: w314 -> [_ w321]
          tunnel: w313 -> [w315 w316]
          tunnel: [w315 w317] -> w312
          frame "Off", Default {
            # "Do nothing"
          }
          frame "Standard" {
            # "Turn the single setpoint into a 3-phase setpoint, take the active DeviceID and send the message"
            n156 = Unbundle By Name(w321) -> ("SCADA Enqueuer"=w318:refnum<class "Message Enqueuer.lvclass">)
            n157 = property on="Channels" class="MCListbox (strict)"() -> ("ItemNames"=w325:string[][], "Value"=w326:i32[])  [unwired: 2 in, 2 out]
            n158 = Index Array(array=w326) -> (element=w327:i32)  [unwired: 1 in]
            n159 = Index Array(array=w325, index (row)=w327, index (col)=3 ("disabled index (col)")) -> (element=w322:string)
            n160 = Bundle By Name(cluster=T15 {"DeviceID"="", "Mode"=enum."Invalid"} ("DER_setGenerationMode"), "Mode"="Gen Mode", "DeviceID"=w322) -> (w319:T15)
            n161 = call "Send Manual Generation Mode Set.vi"("error in (no error)"=w316, "DER_setGenerationMode"=w319, "Message Enqueuer"=w318) -> ("error out"=w317:errorcluster)  [unwired: 7 in, 1 out]
          }
        }
      }
      event "Write Q": Value Change {
        # "#TODO Move some of this code into a message to make sure it only runs while the microgrid is in manual mode"
        # "Set the reactive power setpoint under connected condition"
        n162 = event-data() -> ()  [unwired: 1 in, 1 out]
        n163 = local read "Device Connect"() -> (w331:T3)
        n164 = case "Device Connection Status?" shown="\"Standard\"" w331 {
          tunnel: w330 -> [w332 w335]
          tunnel: [w332 w334] -> w329
          tunnel: w328 -> [_ w337]
          frame "Off", Default {
            # "Do nothing"
          }
          frame "Standard" {
            # "The device is connected, allow the message to go through"
            n165 = property on="Channels" class="MCListbox (strict)"() -> ("ItemNames"=w346:string[][], "Value"=w347:i32[])  [unwired: 2 in, 2 out]
            n166 = Unbundle By Name(w337) -> ("SCADA Enqueuer"=w336:refnum<class "Message Enqueuer.lvclass">)
            n167 = Index Array(array=w347) -> (element=w348:i32)  [unwired: 1 in]
            n168 = Divide(x="Q Setpoint (kVAR)", y=3.0) -> (x/y=w342:dbl)
            n169 = Initialize Array(w342, 3 ("dimension size")) -> (w339:dbl[])
            n170 = Index Array(array=w346, index (row)=w348, index (col)=3 ("disabled index (col)")) -> (element=w340:string)
            n171 = Bundle By Name(cluster=T16 {"DeviceID"="", "ReactivePower (kVAR)"=[]} ("DER_SetPointQ"), "ReactivePower (kVAR)"=w339, "DeviceID"=w340) -> (w333:T16)
            n172 = call "Send Manual Reactive Power Setpoint.vi"("error in (no error)"=w335, "DER_SetPointQ"=w333, "Message Enqueuer"=w336) -> ("error out"=w334:errorcluster)  [unwired: 7 in, 1 out]
          }
        }
      }
      event User Event {
        n173 = event-data() -> ("Device State"=w352:T7, "data"=w351:variant)  [unwired: 1 in]
        n174 = Bundle By Name(cluster=T6 {"Device State"=enum."Invalid", "data"=variant} ("Device State Information"), "Device State"=w352, "data"=w351) -> (w349:T6)
        n175 = Enqueue Element(queue=w350, element=w349) -> ()  [unwired: 2 in, 3 out]
      }
      event User Event {
        # "Handles changes in front panel objects during changes of state."
        n176 = event-data() -> ("Microgrid State"=w355:T10)  [unwired: 1 in]
        n177 = Format Into String(error in=w360, w355) -> (resulting string=→"Current State":string, error out=w359:errorcluster)  [unwired: 2 in]
        n178 = feedback-in #3(w355) -> ()
        n179 = feedback #3() -> (w354:T10)  [unwired: 1 in]
        n180 = case "Microgrid States Switch Statement" shown="\"Discovery\"" w355 {
          tunnel: [u32 16776960 u32 16776960 u32 16744448 u32 255 u32 65280 u32 16711680 u32 8454016 u32 16744576 u32 16776960 u32 16776960 u32 0] -> w361
          tunnel: w359 -> [w373 w383 w401 w413 w423 w436 w445 w455 w464 w473 w476]
          tunnel: [w375 w385 w399 w411 w416 w434 w443 w453 w462 w471 w476] -> w358
          tunnel: w357 -> [_ _ _ _ w417 w428 _ _ _ _ _]
          tunnel: w356 -> [w366 _ _ _ _ _ _ _ _ _ _]
          tunnel: w355 -> [_ _ w395 _ _ _ _ _ _ _ _]
          tunnel: w354 -> [_ _ w394 _ _ _ _ _ _ _ _]
          frame "Discovery" {
            w367 = T17."Disabled and Grayed Out" ("Disabled")
            n181 = Enqueue Element(queue=w366, element=T6 {"Device State"=enum."Clear", "data"=variant}) -> ()  [unwired: 2 in, 3 out]
            n182 = property on="Execution" class="Bool"(error in=w373, "DisabledEnum"=w367, "BoolText.Text"="") -> (error out=w374:errorcluster)  [unwired: 1 in, 1 out]
            n183 = property on="Transition" class="Bool"(error in=w374, "DisabledEnum"=w367, "BoolText.Text"="") -> (error out=w372:errorcluster)  [unwired: 1 in, 1 out]
            n184 = property on="Current Status Bool" class="Bool (strict)"("BoolText.Text"="") -> ()  [unwired: 2 in, 2 out]
            n185 = property on="Start" class="Bool"(error in=w372, "DisabledEnum"=T17."Enabled" ("Disabled"), "BoolText.Text"="Start" ("Boolean Text.Text")) -> (error out=w375:errorcluster)  [unwired: 1 in, 1 out]
          }
          frame "Commissioning" {
            w377 = T17."Disabled and Grayed Out" ("Disabled")
            n186 = property on="Execution" class="Bool"(error in=w383, "DisabledEnum"=w377, "BoolText.Text"="") -> (error out=w384:errorcluster)  [unwired: 1 in, 1 out]
            n187 = property on="Transition" class="Bool"(error in=w384, "DisabledEnum"=w377, "BoolText.Text"="") -> (error out=w382:errorcluster)  [unwired: 1 in, 1 out]
            n188 = property on="Start" class="Bool"(error in=w382, "DisabledEnum"=T17."Enabled" ("Disabled"), "BoolText.Text"="Stop" ("Boolean Text.Text")) -> (error out=w385:errorcluster)  [unwired: 1 in, 1 out]
          }
          frame "Activation" {
            w391 = T17."Disabled and Grayed Out" ("Disabled")
            # "Prevent people from clicking Activate more than once"
            n189 = Equal?(x=w395, y=w394) -> (x = y?=w390:bool)
            n190 = Select(t="", s=w390, f="Activate" ("Boolean Text.Text")) -> (s? t:f=w387:string)
            n191 = Select(t=w391, s=w390, f=T17."Enabled" ("Disabled")) -> (s? t:f=w392:T17)
            n192 = property on="Execution" class="Bool"(error in=w401, "DisabledEnum"=w392, "BoolText.Text"=w387) -> (error out=w402:errorcluster)  [unwired: 1 in, 1 out]
            n193 = property on="Transition" class="Bool"(error in=w402, "DisabledEnum"=w391, "BoolText.Text"="") -> (error out=w400:errorcluster)  [unwired: 1 in, 1 out]
            n194 = property on="Start" class="Bool"(error in=w400, "DisabledEnum"=T17."Enabled" ("Disabled"), "BoolText.Text"="Stop" ("Boolean Text.Text")) -> (error out=w399:errorcluster)  [unwired: 1 in, 1 out]
          }
          frame "Blackstart" {
            n195 = property on="Execution" class="Bool"(error in=w413, "DisabledEnum"=T17."Enabled" ("Disabled"), "BoolText.Text"="Blackstart" ("Boolean Text.Text")) -> (error out=w414:errorcluster)  [unwired: 1 in, 1 out]
            n196 = property on="Transition" class="Bool"(error in=w414, "DisabledEnum"=T17."Disabled and Grayed Out" ("Disabled"), "BoolText.Text"="") -> (error out=w412:errorcluster)  [unwired: 1 in, 1 out]
            n197 = property on="Start" class="Bool"(error in=w412, "DisabledEnum"=T17."Enabled" ("Disabled"), "BoolText.Text"="Stop" ("Boolean Text.Text")) -> (error out=w411:errorcluster)  [unwired: 1 in, 1 out]
          }
          frame "OffGrid" {
            w418 = T17."Enabled" ("Disabled")
            n198 = property on="Execution" class="Bool"(error in=w423, "DisabledEnum"=w418, "BoolText.Text"="Shutdown" ("Boolean Text.Text")) -> (error out=w424:errorcluster)  [unwired: 1 in, 1 out]
            n199 = global read "Global Variables.vi" "Enable Remote Operation"() -> (w415:bool)
            n200 = property on="Transition" class="Bool"(error in=w424, "DisabledEnum"=w418, "BoolText.Text"="Resynchronize" ("Boolean Text.Text")) -> (error out=w422:errorcluster)  [unwired: 1 in, 1 out]
            n201 = property on="Start" class="Bool"(error in=w422, "DisabledEnum"=w418, "BoolText.Text"="Stop" ("Boolean Text.Text")) -> (error out=w416:errorcluster)  [unwired: 1 in, 1 out]
            n202 = case shown="True" w415 {
              tunnel: w417 -> [_ w426]
              frame False {
              }
              frame True {
                n203 = call "Clear Pending Operation in Remote Control.vi"("EMS User Interface in"=w426) -> ()  [unwired: 9 in, 2 out]
              }
            }
          }
          frame "OnGrid" {
            w430 = T17."Enabled" ("Disabled")
            n204 = property on="Execution" class="Bool"(error in=w436, "DisabledEnum"=w430, "BoolText.Text"="Shutdown" ("Boolean Text.Text")) -> (error out=w437:errorcluster)  [unwired: 1 in, 1 out]
            n205 = global read "Global Variables.vi" "Enable Remote Operation"() -> (w427:bool)
            n206 = property on="Transition" class="Bool"(error in=w437, "DisabledEnum"=w430, "BoolText.Text"="Island" ("Boolean Text.Text")) -> (error out=w435:errorcluster)  [unwired: 1 in, 1 out]
            n207 = property on="Start" class="Bool"(error in=w435, "DisabledEnum"=w430, "BoolText.Text"="Stop" ("Boolean Text.Text")) -> (error out=w434:errorcluster)  [unwired: 1 in, 1 out]
            n208 = case shown="True" w427 {
              tunnel: w428 -> [_ w438]
              frame False {
              }
              frame True {
                n209 = call "Clear Pending Operation in Remote Control.vi"("EMS User Interface in"=w438) -> ()  [unwired: 9 in, 2 out]
              }
            }
          }
          frame "Island" {
            w439 = T17."Disabled and Grayed Out" ("Disabled")
            n210 = property on="Execution" class="Bool"(error in=w445, "DisabledEnum"=w439, "BoolText.Text"="") -> (error out=w446:errorcluster)  [unwired: 1 in, 1 out]
            n211 = property on="Transition" class="Bool"(error in=w446, "DisabledEnum"=w439, "BoolText.Text"="") -> (error out=w444:errorcluster)  [unwired: 1 in, 1 out]
            n212 = property on="Start" class="Bool"(error in=w444, "DisabledEnum"=w439, "BoolText.Text"="") -> (error out=w443:errorcluster)  [unwired: 1 in, 1 out]
          }
          frame "Resynchronization" {
            w449 = T17."Disabled and Grayed Out" ("Disabled")
            n213 = property on="Execution" class="Bool"(error in=w455, "DisabledEnum"=w449, "BoolText.Text"="") -> (error out=w456:errorcluster)  [unwired: 1 in, 1 out]
            n214 = property on="Transition" class="Bool"(error in=w456, "DisabledEnum"=w449, "BoolText.Text"="") -> (error out=w454:errorcluster)  [unwired: 1 in, 1 out]
            n215 = property on="Start" class="Bool"(error in=w454, "DisabledEnum"=w449, "BoolText.Text"="") -> (error out=w453:errorcluster)  [unwired: 1 in, 1 out]
          }
          frame "Shutdown" {
            w458 = T17."Disabled and Grayed Out" ("Disabled")
            n216 = property on="Execution" class="Bool"(error in=w464, "DisabledEnum"=w458, "BoolText.Text"="") -> (error out=w465:errorcluster)  [unwired: 1 in, 1 out]
            n217 = property on="Transition" class="Bool"(error in=w465, "DisabledEnum"=w458, "BoolText.Text"="") -> (error out=w463:errorcluster)  [unwired: 1 in, 1 out]
            n218 = property on="Start" class="Bool"(error in=w463, "DisabledEnum"=w458, "BoolText.Text"="") -> (error out=w462:errorcluster)  [unwired: 1 in, 1 out]
          }
          frame "Stop" {
            w467 = T17."Disabled and Grayed Out" ("Disabled")
            n219 = property on="Execution" class="Bool"(error in=w473, "DisabledEnum"=w467, "BoolText.Text"="") -> (error out=w474:errorcluster)  [unwired: 1 in, 1 out]
            n220 = property on="Transition" class="Bool"(error in=w474, "DisabledEnum"=w467, "BoolText.Text"="") -> (error out=w472:errorcluster)  [unwired: 1 in, 1 out]
            n221 = property on="Start" class="Bool"(error in=w472, "DisabledEnum"=w467, "BoolText.Text"="") -> (error out=w471:errorcluster)  [unwired: 1 in, 1 out]
          }
          frame "Manual" {
          }
        }
        n222 = property on="Current State" class="Str"(error in=w358, "Text.BGColor"=w361) -> (error out=w362:errorcluster)  [unwired: 1 in, 1 out]
      }
      event User Event {
        # "Simply updates the Current Status FP object visible in Automatic Mode"
        n223 = event-data() -> ("Current Status"=w477:string)  [unwired: 1 in]
        n224 = property on="Current Status Bool" class="Bool (strict)"("BoolText.Text"=w477) -> ()  [unwired: 2 in, 2 out]
      }
      event User Event {
        # "Find current deviceID in updated list of devices"
        # "Get deviceID for currently selected device"
        # "Callback to set the ItemNames within the Device List"
        n225 = event-data() -> ("Item Names"=w485:string[][])  [unwired: 1 in]
        n226 = property on="Channels" class="MCListbox (strict)"(error in=w491) -> (error out=w490:errorcluster, "Value"=w487:i32[], "ItemNames"=w489:string[][])  [unwired: 1 in, 1 out]
        n227 = Index Array(array=w487) -> (element=w486:i32)  [unwired: 1 in]
        n228 = Index Array(array=w489, index (row)=w486, index (col)=3 ("disabled index (col)")) -> (element=w482:string)
        n229 = property on="Channels" class="MCListbox (strict)"(error in=w490, "ItemNames"=w485) -> (error out=w480:errorcluster)  [unwired: 1 in, 1 out]
        n230 = Index Array(array=w485, index (col)=3 ("disabled index (col)")) -> (element=w483:string[])  [unwired: 1 in]
        n231 = Search 1D Array(1D array=w483, element=w482) -> (index of element=w479:i32)  [unwired: 1 in]
        n232 = Greater Or Equal To 0?(x=w479) -> (x >= 0?=w481:bool)
        n233 = case shown="True" w481 {
          tunnel: w480 -> [w493 w502]
          tunnel: w479 -> [_ w501]
          tunnel: [w492 w499] -> w478
          frame False {
            # "Previously selected device not found in list"
            n234 = local read "Connect"() -> (w494:bool)
            n235 = case shown="True" w494 {
              tunnel: w493 -> [w495 w497]
              tunnel: [w495 w496] -> w492
              frame False {
                # "Not connected.  Do nothing."
              }
              frame True {
                # "Send disconnect"
                n236 = property on="Connect" class="Bool (strict)"(error in=w497, "Val(Sgnl)"=FALSE ("Connect")) -> (error out=w496:errorcluster)  [unwired: 1 in, 1 out]
              }
            }
          }
          frame True {
            # "Current DeviceID found in updated list.  Ensure it stays highlighted.  This is NOT a value signaling property, so it should NOT attempt to connect/disconnect"
            n237 = Build Array(w501) -> (w500:i32[])
            n238 = property on="Channels" class="MCListbox (strict)"(error in=w502, "Value"=w500) -> (error out=w499:errorcluster)  [unwired: 1 in, 1 out]
          }
        }
      }
      event User Event {
        # "Callback that updates Real Power Measurements visible in Manual Control Mode."
        n239 = event-data() -> ("P Meas"=→"P Meas":dbl[])  [unwired: 1 in]
      }
      event User Event {
        # "Callback that updates Reactive Power Measurements visible in Manual Control Mode."
        n240 = event-data() -> ("Q Meas"=→"Q Meas":dbl[])  [unwired: 1 in]
      }
      event User Event {
        # "Callback used when device under manual control connects to limit Real Power input to device limits."
        n241 = event-data() -> ("Scale.Range:Maximum"=w507:dbl)  [unwired: 1 in]
        n242 = property on="P Setpoint (kW)" class="Slide (strict)"(error in=w506, "Scale.Maximum"=w507) -> (error out=w505:errorcluster)  [unwired: 1 in, 1 out]
      }
      event User Event {
        # "Callback used when device under manual control connects to limit Reactive Power input to device limits."
        n243 = event-data() -> ("Scale.Range:Maximum"=w509:dbl)  [unwired: 1 in]
        n244 = property on="Q Setpoint (kVAR)" class="Slide (strict)"(error in=w510, "Scale.Maximum"=w509) -> (error out=w508:errorcluster)  [unwired: 1 in, 1 out]
      }
      event User Event {
        # "Callback to display activation status to the user in Manual Control mode"
        n245 = event-data() -> ("Active"=→"Active":bool, "Inactive"=→"Inactive":bool)  [unwired: 1 in]
      }
      event Panel Close? {
        # "Trying to close the panel will casue the application to stop first."
        n246 = event-data() -> ()  [unwired: 1 in, 1 out]
        n247 = Unbundle By Name(w519) -> ("SCADA Enqueuer"=w518:refnum<class "Message Enqueuer.lvclass">)
        n248 = call <vilib>:"Send Normal Stop.vi"("Message Enqueuer"=w517) -> ("error out"=w514:errorcluster)  [unwired: 10 in]
        n249 = call <vilib>:"Send Normal Stop.vi"("Message Enqueuer"=w518) -> ("error out"=w515:errorcluster)  [unwired: 10 in]
        n250 = Merge Errors(w516, w515, w514) -> (w513:errorcluster)
        n251 = event-data("Discard?"=TRUE) -> ()  [unwired: 1 in, 1 out]
      }
    }
    n252 = Or(x=w69, y=w68) -> (x .or. y?=w67:bool)
  }
  n253 = while {
    tunnel: w11 -> [w529]
    tunnel: w10 -> [w525]
    shift-right: [w524] -> _
    shift-left: T1[] [] ("Array") -> [w523]
    tunnel: w2 -> [w522]
    stop <- w526 stop-if-true
    # "This loop is solely responsible for updating the device information on the front panel"
    n254 = Dequeue Element(queue=w529) -> (element=w527:T6, error out=w528:errorcluster)  [unwired: 2 in, 2 out]
    n255 = case shown="No Error" w528 {
      tunnel: w527 -> [w536 _]
      tunnel: [_ TRUE] -> w526
      tunnel: w525 -> [w533 _]
      tunnel: [w532 w638] -> w524
      tunnel: w523 -> [w531 w638]
      tunnel: w522 -> [w530 _]
      frame No Error {
        n256 = Unbundle By Name(w536) -> ("Device State"=w535:T7, "data"=w534:variant)
        n257 = case shown="\"Update DER_Measurement\"" w535 {
          selector: w535 -> [_ _ _ w572 _ _ _ _]
          tunnel: w534 -> [_ _ w563 w576 w595 w623 w629 w637]
          tunnel: w533 -> [_ w541 w564 w574 w593 w621 w627 w635]
          tunnel: [w537 _ w562 w573 w592 w619 w626 w633] -> w532
          tunnel: w531 -> [w537 w542 w561 w573 w592 w619 w626 w633]
          tunnel: w530 -> [_ _ _ _ w590 w618 w624 w632]
          frame "Invalid" {
          }
          frame "Clear" {
            # "Clear all data and colors from the Devices listbox"
            n258 = property class="MCListbox (strict)"(reference=w541) -> ("ColHdrString"=w540:string[])  [unwired: 1 in, 2 out]
            n259 = Array Size(array=w540) -> (size(s)=w539:i32)
            n260 = for {
              shift-right: [w550] -> w543
              shift-left: _ -> [w551]
              shift-right: [w549] -> w544
              shift-left: w541 -> [w547]
              tunnel: w542 -> [_] mode=indexing
              tunnel: w539 -> [w546]
              i -> [w548]
              n261 = for {
                N: w546 -> [_]
                tunnel: w551 -> [w559]
                tunnel: [w558] -> w550
                shift-right: [w556] -> w549
                shift-left: w547 -> [w560]
                tunnel: w548 -> [w554]
                i -> [w552]
                n262 = Bundle By Name(cluster=T19 {"Row"=0, "Column"=0} ("Active Cell:Active Cell"), "Row"=w554, "Column"=w552) -> (w553:T19)
                n263 = property on="Property Node" class="MCListbox (strict)"(reference=w560, error in=w559, "ActiveCell"=w553, "CellBG"=u32 16777215) -> (reference out=w556:refnum<vi>, error out=w558:errorcluster)
              }
            }
            n264 = property class="MCListbox (strict)"(reference=w544, error in=w543, "Value"=-1, "ItemNames"=string[][] [] ("Item Names")) -> ()  [unwired: 2 out]
          }
          frame "DevIDs in Config" {
            n265 = Variant To Data(type=w561, Variant=w563) -> (data=w562:T1[])  [unwired: 1 in, 1 out]
            n266 = call "Initialize Listbox.vi"("Expected DevIDs"=w562, "MulticolumnListbox in"=w564) -> ()  [unwired: 8 in, 2 out]
          }
          frame "DevIDs on uGrid", "DevIDs not on uGrid" {
            n267 = Equal?(x=w572, y=Device_State."DevIDs on uGrid") -> (x = y?=w565:bool)
            n268 = Variant To Data(type=w573, Variant=w576) -> (data=w575:T1[])  [unwired: 1 in, 1 out]
            n269 = Select(t=u32 0, s=w565, f=u32 13816530) -> (s? t:f=w568:u32)
            n270 = for {
              tunnel: w575 -> [w582] mode=indexing
              tunnel: w573 -> [w585]
              tunnel: [w584] -> _
              tunnel: w568 -> [w581]
              tunnel: [w580] -> w567 mode=indexing
              shift-right: [w579] -> w566
              shift-left: w574 -> [w583]
              # "Update text color to indicate domain presence of device"
              n271 = Search 1D Array(1D array=w585, element=w582) -> (index of element=w580:i32)  [unwired: 1 in]
              n272 = Bundle By Name(cluster=T19 {"Row"=0, "Column"=0} ("Active Cell:Active Cell"), "Row"=w580) -> (w586:T19)
              n273 = property class="MCListbox (strict)"(reference=w583, "ActiveCell"=w586, "CellFontColor"=w581) -> (reference out=w579:refnum<vi>, error out=w584:errorcluster)  [unwired: 1 in]
            }
            n274 = case shown="False" w565 {
              tunnel: w567 -> [w578 _]
              tunnel: w566 -> [w577 _]
              frame False {
                n275 = call "Partial Clear of Row in Listbox.vi"("Rows to Clear"=w578, "MulticolumnListbox in"=w577) -> ()  [unwired: 10 in]
              }
              frame True {
              }
            }
          }
          frame "Update IED_Status" {
            n276 = Unbundle By Name(w590) -> ("Active Column"=w589:i32, "Inactive Column"=w588:i32)
            n277 = Variant To Data(type=T20[] [] ("Array"), Variant=w595) -> (data=w591:T20[])  [unwired: 1 in, 1 out]
            n278 = for {
              tunnel: [w607] -> _ mode=indexing
              tunnel: w592 -> [w606]
              tunnel: w591 -> [w603] mode=indexing
              tunnel: w593 -> [w604]
              tunnel: w589 -> [w597]
              tunnel: w588 -> [w596]
              # "Green background signifies boolean is True"
              n279 = Unbundle By Name(w603) -> ("DeviceID"=w602:T1, "Active"=w600:bool, "Inactive"=w599:bool)
              n280 = Search 1D Array(1D array=w606, element=w602) -> (index of element=w605:i32)  [unwired: 1 in]
              n281 = Build Array(w600, w599) -> (w601:bool[])
              n282 = Build Array(w597, w596) -> (w598:i32[])
              n283 = for {
                tunnel: [w615] -> w607
                tunnel: w605 -> [w614]
                tunnel: w604 -> [w613]
                tunnel: w601 -> [w612] mode=indexing
                tunnel: w598 -> [w608] mode=indexing
                n284 = Bundle By Name(cluster=T19 {"Row"=0, "Column"=0} ("Active Cell:Active Cell"), "Row"=w614, "Column"=w608) -> (w616:T19)
                n285 = Select(t=u32 65280, s=w612, f=u32 16777215) -> (s? t:f=w609:u32)
                n286 = property on="Property Node" class="MCListbox (strict)"(reference=w613, "ActiveCell"=w616, "CellBG"=w609) -> (error out=w615:errorcluster)  [unwired: 1 in, 1 out]
              }
            }
          }
          frame "Update DER_Measurement" {
            n287 = Variant To Data(type=T22[] [] ("Array"), Variant=w623) -> (data=w620:T22[])  [unwired: 1 in, 1 out]
            n288 = call "Update DER_Measurement in Listbox.vi"("DevIDs in Config"=w619, "Listbox Columns"=w618, "DER_Measurement (Array)"=w620, "MulticolumnListbox in"=w621) -> ()  [unwired: 8 in]
          }
          frame "Update SmartRelay_Measurement" {
            n289 = Variant To Data(type=T23[] [] ("Array"), Variant=w629) -> (data=w625:T23[])  [unwired: 1 in, 1 out]
            n290 = call "Update SmartRelay_Measurement in Listbox.vi"("DevIDs in Config"=w626, "Listbox Columns"=w624, "SmartRelay_Measurement (Array)"=w625, "MulticolumnListbox in"=w627) -> ()  [unwired: 8 in]
          }
          frame "Update DER_Status" {
            n291 = Variant To Data(type=T24[] [] ("Array"), Variant=w637) -> (data=w634:T24[])  [unwired: 1 in, 1 out]
            n292 = Unbundle By Name(w632) -> ("VF Column"=w631:i32, "Modes Column"=w630:i32)
            n293 = call "Update DER_Status in Listbox.vi"("Mode Column"=w630, "VF Column"=w631, "DevIDs in Config"=w633, "DER_Status (Array)"=w634, "MulticolumnListbox in"=w635) -> ()  [unwired: 7 in]
          }
        }
      }
      frame Error {
      }
    }
    "DevIDs in Config" <- w523
  }
  n294 = call-parent "Actor Core.vi"("error in"=w14, "Actor in"=w15) -> ("error out"=w29:errorcluster, "Actor out"=→"Actor out":refnum<class "Actor.lvclass">)  [unwired: 8 in]
  n295 = Unregister For Events(event registration refnum=w49) -> (error out=w12:errorcluster)  [unwired: 1 in]
  n296 = call-dynamic "Error Handler.vi"("error in"=w23, "EMS Generic in"=w15) -> ("error out"=w22:errorcluster, "EMS Generic out"=w21:refnum<class "EMS User Interface.lvclass">)  [unwired: 8 in]
  n297 = Release Queue(queue=w11, error in (no error)=w12) -> ()  [unwired: 1 in, 3 out]
  n298 = call-dynamic "Destroy User Events.vi"("error in"=w22, "Master Controller in"=w21) -> ("error out"=w28:errorcluster)  [unwired: 8 in, 1 out]
  n299 = call "Status Update.vi"("Command (Write)"=Status_Message_Command."Kill", "error in"=w28, "Status Update"="") -> ("error out"=w24:errorcluster)  [unwired: 7 in, 1 out]
  n300 = Merge Errors(w24, w29) -> (w26:errorcluster)
  n301 = call <vilib>:"Simple Error Handler.vi"("error in (no error)"=w26) -> ("error out"=→"error out":errorcluster)  [unwired: 4 in, 4 out]
